vi "Configure Trigger (Video).vi"(0 "VISA resource name":refnum<visa-resource-name>, 1 "Video Line Number (1)":i16=1, 2 "Custom Line Period (6.36E-5)":dbl=6.36e-05, 3 "Custom Sync Interval (4.7E-6)":dbl=4.7e-06, 5 "Source (0:Channel1)":u16(ring) items=["Channel1", "Channel2", "Channel3", "Channel4"], 7 "Polarity (0:Normal)":u16(ring) items=["Normal", "Inverted"], 9 "Trigger On (2:All Fields)":u16(ring)=2 items=["Odd", "Even", "All Fields", "All Lines", "Line"], 11 "error in (no error)":errorcluster, 12 "Holdoff By Fields (0.0)":dbl, 13 "Format (NTSC)":u16(ring) items=["NTSC", "PAL", "SECAM", "HD480P60", "HD576P50", "HD720P30", "HD720P50", "HD720P60", "HD1080I50", "HD1080I60", "HD1080P24", "HD1080P25", "HD1080P30", "HD1080P50", "HD1080P60", "HD1080SF24", "BiLevel", "TriLevel"]) -> (4 "VISA resource name out":refnum<visa-resource-name>, 15 "error out":errorcluster)   [LabVIEW 2015, in "Tektronix 7000 Series.lvlib"]
doc: "Configures Video trigger settings for an oscilloscope.\n\n<B>Note:</B> \nTDS6000, TDS6000B, TDS6000C ,TDS7000, CSA7000, CSA7000B, TDS7000B, DPO70000 and DSA 70000 series oscilloscopes don't support Video Trigger."
uses:
  <instrlib>/Tektronix 7000 Series/Tektronix 7000 Series.lvlib
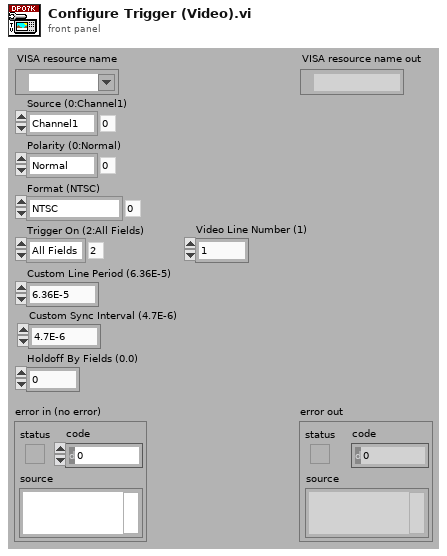
[diagram p1: front panel]
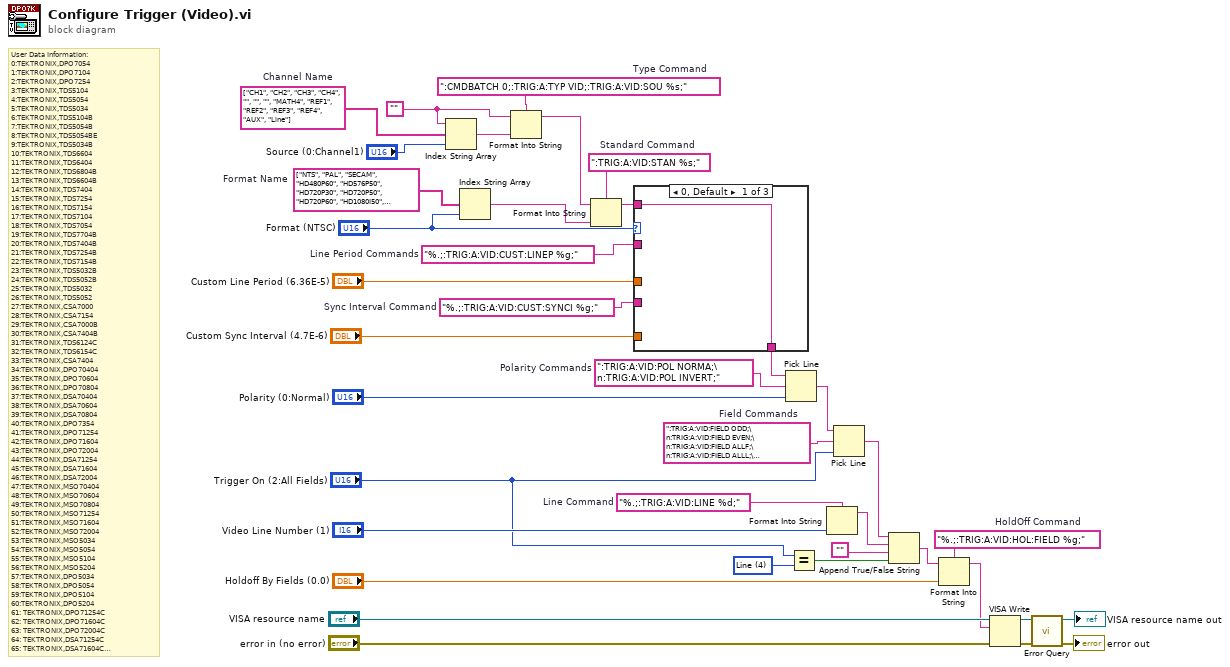
[diagram p0: block diagram]
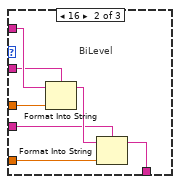
[diagram p2: hidden frame]
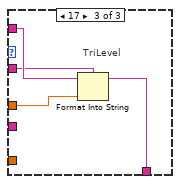
[diagram p3: hidden frame]
diagram:
  w14 = "%.;:TRIG:A:VID:HOL:FIELD %g;"  # HoldOff Command
  w21 = u16 4 items=["Odd", "Even", "All Fields", "All Lines", "Line"] ("Trigger On (2:All Fields)")
  w22 = "%.;:TRIG:A:VID:LINE %d;"  # Line Command
  w23 = ":TRIG:A:VID:FIELD ODD;\n:TRIG:A:VID:FIELD EVEN;\n:TRIG:A:VID:FIELD ALLF;\n:TRIG:A:VID:FIELD ALLL;\n:TRIG:A:VID:FIELD NUMER;"  # Field Commands
  w26 = ":TRIG:A:VID:POL NORMA;\n:TRIG:A:VID:POL INVERT;"  # Polarity Commands
  w28 = "%.;:TRIG:A:VID:CUST:SYNCI %g;"  # Sync Interval Command
  w2 = "%.;:TRIG:A:VID:CUST:LINEP %g;"  # Line Period Commands
  w30 = ":TRIG:A:VID:STAN %s;"  # Standard Command
  w33 = string[] ["NTS", "PAL", "SECAM", "HD480P60", "HD576P50", "HD720P30", "HD720P50", "HD720P60", "HD1080I50", "HD1080I60", "HD1080P24", "HD1080P25", "HD1080P30", "HD1080P50", "HD1080P60", "HD1080SF24", "BIL", "TRIL"]  # Format Name
  w36 = ":CMDBATCH 0;:TRIG:A:TYP VID;:TRIG:A:VID:SOU %s;"  # Type Command
  w38 = string[] ["CH1", "CH2", "CH3", "CH4", "", "", "", "MATH4", "REF1", "REF2", "REF3", "REF4", "AUX", "Line"]  # Channel Name
  w34 = ""
  # "User Data Information:\n0:TEKTRONIX,DPO7054\n1:TEKTRONIX,DPO7104\n2:TEKTRONIX,DPO7254\n3:TEKTRONIX,TDS5104\n4:TEKTRONIX,TDS5054\n5:TEKTRONIX,TDS5034\n6:TEKTRONIX,TDS5104B\n7:TEKTRONIX,TDS5054B\n8:TEKTRONIX,TDS5054BE\n9:TEKTRONIX,TDS5034B\n10:TEKTRONIX,TDS6604\n11:TEKTRONIX,TDS6404\n12:TEKTRONIX,TDS6804B\n13:TEKTRONIX,TDS6604B\n14:TEKTRONIX,TDS7404\n15:TEKTRONIX,TDS7254\n16:TEKTRONIX,TDS7154\n17:TEKTRONIX,TDS7104\n18:TEKTRONIX,TDS7054\n19:TEKTRONIX,TDS7704B\n20:TEKTRONIX,TDS7404B\n21:TEKTRONIX,TDS7254B\n22:TEKTRONIX,TDS7154B\n23:TEKTRONIX,TDS5032B\n24:TEKTRONIX,TDS5052B\n25:TEKTRONIX,TDS5032\n26:TEKTRONIX,TDS5052\n27:TEKTRONIX,CSA7000\n28:TEKTRONIX,CSA7154\n29:TEKTRONIX,CSA7000B\n30:TEKTRONIX,CSA7404B\n31:TEKTRONIX,TDS6124C\n32:TEKTRONIX,TDS6154C\n33:TEKTRONIX,CSA7404\n34:TEKTRONIX,DPO70404\n35:TEKTRONIX,DPO70604\n36:TEKTRONIX,DPO70804\n37:TEKTRONIX,DSA70404\n38:TEKTRONIX,DSA70604\n39:TEKTRONIX,DSA70804\n40:TEKTRONIX,DPO7354\n41:TEKTRONIX,DPO71254\n42:TEKTRONIX,DPO71604\n43:TEKTRONIX,DPO72004\n44:TEKTRONIX,DSA71254\n45:TEKTRONIX,DSA71604\n46:TEKTRONIX,DSA72004\n47:TEKTRONIX,MSO70404\n48:TEKTRONIX,MSO70604\n49:TEKTRONIX,MSO70804\n50:TEKTRONIX,MSO71254\n51:TEKTRONIX,MSO71604\n52:TEKTRONIX,MSO72004\n53:TEKTRONIX,MSO5034\n54:TEKTRONIX,MSO5054\n55:TEKTRONIX,MSO5104\n56:TEKTRONIX,MSO5204\n57:TEKTRONIX,DPO5034\n58:TEKTRONIX,DPO5054\n59:TEKTRONIX,DPO5104\n60:TEKTRONIX,DPO5204\n61: TEKTRONIX,DPO71254C\n62: TEKTRONIX,DPO71604C\n63: TEKTRONIX,DPO72004C\n64: TEKTRONIX,DSA71254C\n65: TEKTRONIX,DSA71604C\n66: TEKTRONIX,DSA72004C\n67: TEKTRONIX,MSO71254C\n68: TEKTRONIX,MSO71604C\n69: TEKTRONIX,MSO72004C"
  n1 = Index String Array(1:"Source (0:Channel1)", 2:w38, 3:w34) -> (0:w35:string)
  n2 = Index String Array(1:"Format (NTSC)", 2:w33) -> (0:w31:string)  [unwired: 1 in]
  n3 = Format Into String(format string=w36, initial string=w34, w35) -> (resulting string=w32:string)  [unwired: 1 in, 1 out]
  n4 = Format Into String(format string=w30, initial string=w32, w31) -> (resulting string=w29:string)  [unwired: 1 in, 1 out]
  n5 = case shown="0, Default" "Format (NTSC)" {
    tunnel: w29 -> [w39 w46 w50]
    tunnel: "Custom Line Period (6.36E-5)" -> [_ w44 w48]
    tunnel: w28 -> [_ w42 _]
    tunnel: [w39 w40 w47] -> w27
    tunnel: w2 -> [_ w45 w49]
    tunnel: "Custom Sync Interval (4.7E-6)" -> [_ w41 _]
    frame 0, Default {
    }
    frame 16 {
      # "BiLevel"
      n6 = Format Into String(format string=w45, initial string=w46, w44) -> (resulting string=w43:string)  [unwired: 1 in, 1 out]
      n7 = Format Into String(format string=w42, initial string=w43, w41) -> (resulting string=w40:string)  [unwired: 1 in, 1 out]
    }
    frame 17 {
      # "TriLevel"
      n8 = Format Into String(format string=w49, initial string=w50, w48) -> (resulting string=w47:string)  [unwired: 1 in, 1 out]
    }
  }
  n9 = Pick Line(string ("")=w27, multi-line string=w26, line index="Polarity (0:Normal)") -> (output string=w24:string)
  n10 = Equal?(x="Trigger On (2:All Fields)", y=w21) -> (x = y?=w19:bool)
  n11 = Format Into String(format string=w22, "Video Line Number (1)") -> (resulting string=w18:string)  [unwired: 2 in, 1 out]
  n12 = Pick Line(string ("")=w24, multi-line string=w23, line index="Trigger On (2:All Fields)") -> (output string=w17:string)
  n13 = Append True/False String(1:w19, 2:"", 3:w18, 4:w17) -> (0:w15:string)
  n14 = Format Into String(format string=w14, initial string=w15, "Holdoff By Fields (0.0)") -> (resulting string=w8:string)  [unwired: 1 in, 1 out]
  n15 = VISA Write(VISA resource name="VISA resource name", write buffer=w8, error in (no error)="error in (no error)") -> (VISA resource name out=w12:refnum<visa-resource-name>, error out=w11:errorcluster)  [unwired: 1 out]
  n16 = call <instrlib>:"Error Query.vi"("error in (no error)"=w11, "VISA resource name"=w12) -> ("error out"=→"error out":errorcluster, "VISA resource name out"=→"VISA resource name out":refnum<visa-resource-name>)  [unwired: 6 in, 2 out]
